vi "DIAdem Close Reference.vi"(8 "error in (no error)":errorcluster, 11 "DIAdem Reference":T1) -> (0 "error out":errorcluster)   [LabVIEW 2017]
doc: "This VI closes the reference to the DIAdem application. The DIAdem environment is closed if it was not originally open."
uses:
  <vilib>/ExportToExcel/DIAdem Reference.ctl
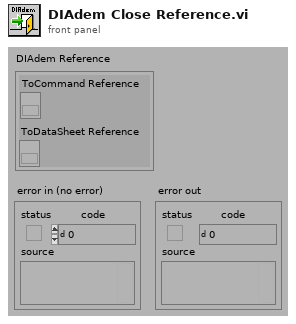
[diagram p1: front panel]
types:
  T1 = typedef "DIAdem Reference.ctl" = cluster{"ToCommand Reference":refnum<k7>, "ToDataSheet Reference":refnum<k7>}
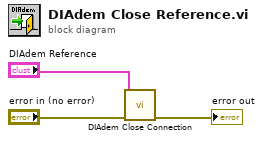
[diagram p0: block diagram]
diagram:
  n1 = call <vilib>:"DIAdem Close Connection.vi"("error in (no error)"="error in (no error)", "DIAdem Reference"="DIAdem Reference") -> ("error out"=→"error out":errorcluster)  [unwired: 9 in]
